vi "Menu.vi"() -> (0 "result":i32)   [LabVIEW 2021]
doc: "Este VI permite escojer el nivel que deseamos jugar..."
panel:
  in  "Cluster":T1
  # "WYBIERZ POZIOM"
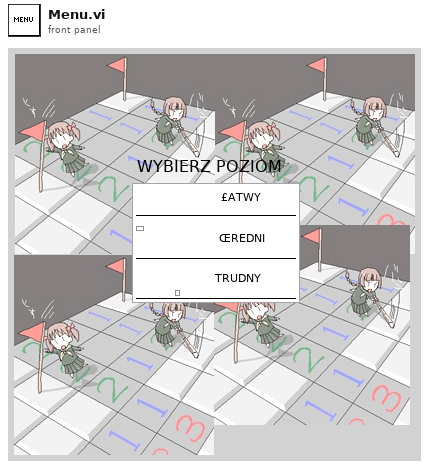
[diagram p1: front panel]
types:
  T1 = cluster{"Log 4":bool, "Log 9":bool, "Log 13":bool}
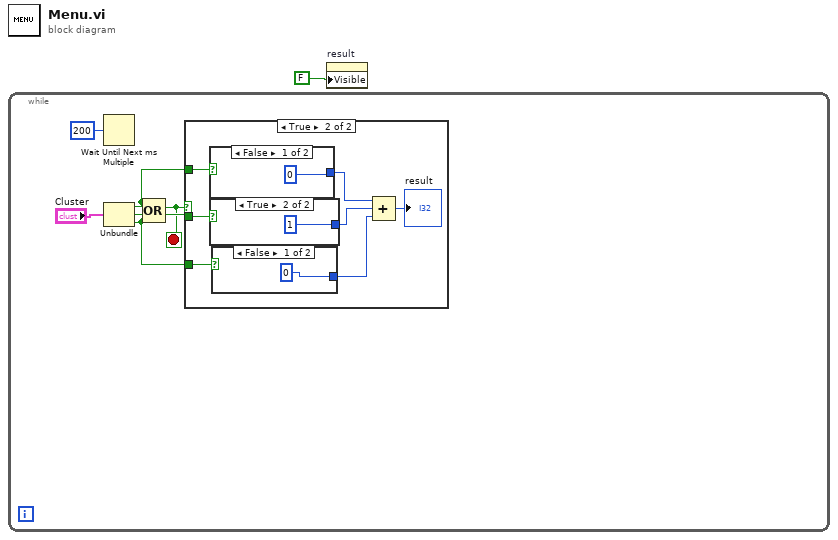
[diagram p0: block diagram]
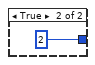
[diagram p3: hidden frame]
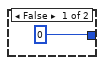
[diagram p4: hidden frame]
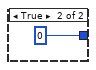
[diagram p5: hidden frame]
diagram:
  n1 = while {
    stop <- w3 stop-if-true
    n2 = Wait Until Next ms Multiple(millisecond multiple=u32 200) -> ()  [unwired: 1 out]
    n3 = Unbundle("Cluster") -> ("Log 4"=w6:bool, "Log 9"=w5:bool, "Log 13"=w4:bool)
    n4 = Compound Arithmetic op=OR(w6, w5, w4) -> (w3:bool)
    n5 = case shown="True" w3 {
      tunnel: w6 -> [_ w14]
      tunnel: w5 -> [_ w13]
      tunnel: w4 -> [_ w12]
      frame False {
      }
      frame True {
        n6 = case shown="False" w14 {
          tunnel: [0 0] -> w11
          frame False {
          }
          frame True {
          }
        }
        n7 = case shown="True" w13 {
          tunnel: [0 1] -> w10
          frame False {
          }
          frame True {
          }
        }
        n8 = case shown="False" w12 {
          tunnel: [0 2] -> w9
          frame False {
          }
          frame True {
          }
        }
        n9 = Compound Arithmetic op=ADD(w11, w10, w9) -> (→"result":i32)
      }
    }
  }
  n10 = property on="result" class="DigNum (strict)"("Visible"=FALSE) -> ()  [unwired: 2 in, 2 out]
